vi "Register Track.vi"(6 "Track ID":u64, 7 "Track Name":string, 8 "error in":errorcluster) -> (0 "error out":errorcluster)   [LabVIEW 2024, in "VS Tracing API.lvlib"]
doc: "Creates a custom track that can be used for recording events outside timed structures.\nThe created track appears as a separate timeline in the trace and can be used with <i>Event Start On Track</i> and <i>Event Stop On Track</i>.\n\n<b>Parameters</b>\n• <b>Track ID</b>: Unique identifier for the track. This value must be unique within the trace session.\n• <b>Track Name</b>: Display name of the track shown in trace.\n\n<b>Notes</b>\n• The Track ID can be any user-defined unique value.\n• A track must be registered before events can be recorded on it."
uses:
  VS Tracing API.lvlib
  libvs_perfetto.dll
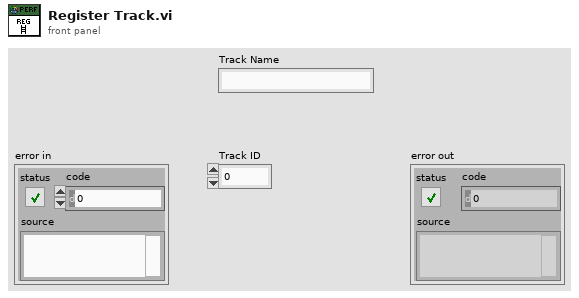
[diagram p1: front panel]
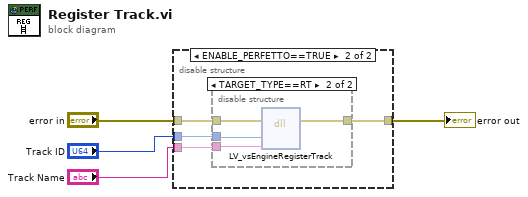
[diagram p0: block diagram]
diagram:
  n1 = disable-structure shown="ENABLE_PERFETTO==TRUE" {
    disable-tunnel: "Track Name" -> [_ w7]
    disable-tunnel: "error in" -> [w5 w8]
    disable-tunnel: [w5 w9] -> w3
    disable-tunnel: "Track ID" -> [_ w6]
    frame condition #0 (active) {
    }
    frame condition #1 {
      n2 = disable-structure shown="TARGET_TYPE==RT" {
        disable-tunnel: [w10 w14] -> w9
        disable-tunnel: w8 -> [w10 w13]
        disable-tunnel: w7 -> [_ w12]
        disable-tunnel: w6 -> [_ w11]
        frame condition #0 (active) {
        }
        frame condition #1 {
          n3 = dll-call lib="libvs_perfetto.*" fn="LV_vsEngineRegisterTrack"(error in=w13, "trackId"=w11, "trackName"=w12) -> (error out=w14:errorcluster)  [unwired: 5 in, 1 out]
        }
      }
    }
  }
  "error out" <- w3
